vi "Load from Text File.vi"(8 "error in":errorcluster, 11 "JSON in":refnum<class "JSON.lvclass">) -> (0 "error out":errorcluster, 2 "text":string, 3 "JSON out":refnum<class "JSON.lvclass">)   [LabVIEW 2017, in "Reports.lvlib" / "JSON.lvclass"]
doc: "This method serves for \nread string from external\ntext file"
uses:
  JSON.lvclass
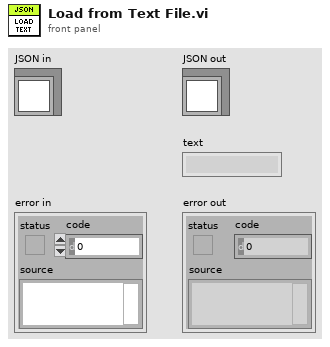
[diagram p1: front panel]
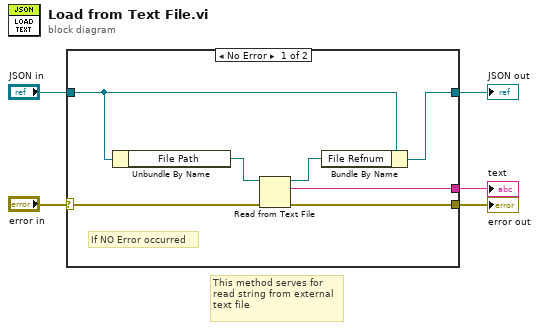
[diagram p0: block diagram]
diagram:
  # "This method serves for \nread string from external\ntext file"
  n1 = case shown="No Error" "error in" {
    selector: "error in" -> [w11 w14]
    tunnel: [w10 w14] -> w4
    tunnel: [w7 w13] -> w2
    tunnel: "JSON in" -> [w8 w13]
    tunnel: [w6 _] -> w1
    frame No Error {
      # "If NO Error occurred"
      n2 = Unbundle By Name(w8) -> ("File Path"=w12:path)
      n3 = Read from Text File(file (use dialog)=w12, error in=w11) -> (refnum out=w9:refnum<file>, text=w6:string, error out=w10:errorcluster)  [unwired: 2 in, 1 out]
      n4 = Bundle By Name(cluster=w8, "File Refnum"=w9) -> (w7:refnum<class "JSON.lvclass">)
    }
    frame Error {
    }
  }
  "error out" <- w4
  "JSON out" <- w2
  "text" <- w1
